vi "Example_LVQ.vi"() -> ()   [LabVIEW 2009]
uses:
  <vilib>/addons/Machine Learning/Utilities/Riffle (matrix with labels).vi
  <vilib>/addons/Machine Learning/NILabs_MLT.lvlib
panel:
  out "Data and learned centroids":cluster{"X":dbl[], "Y":dbl[]}[](graph)
  in  "# of samples":i32=1000
  in  "Parameters":cluster{"learning rate":dbl, "da":dbl}={"learning rate"=0.1, "da"=0.9}
  in  "stopping criteria":cluster{"tolarence":dbl, "max iterations":i32}={"tolarence"=1e-05, "max iterations"=50}
  in  "# of neurons":i32=16
  out "Time (ms)":u32
  # "Introduction:\nLearning Vector Quantization (LVQ) is used to learn the cluster structure of a data distrubution with four Gaussian centers."
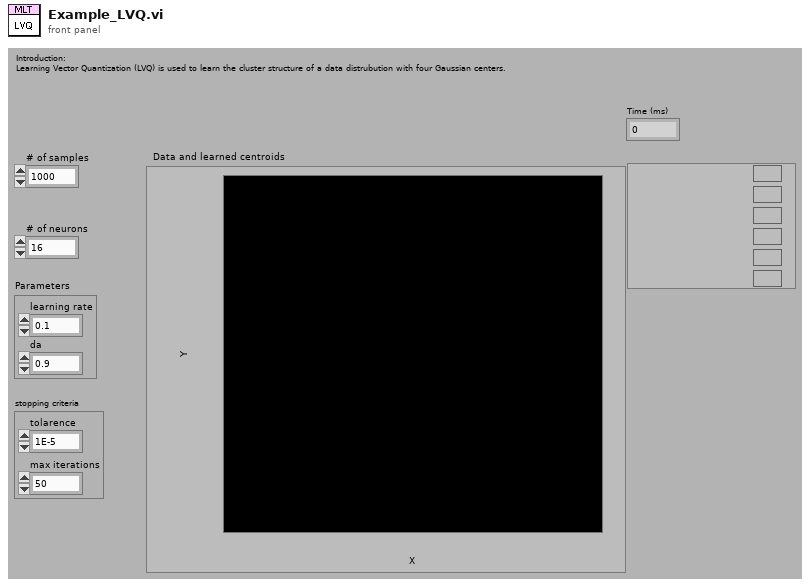
[diagram p1: front panel]
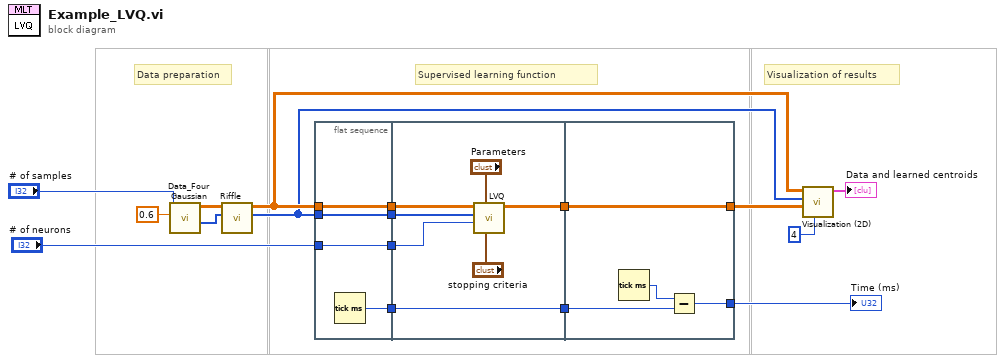
[diagram p0: block diagram]
diagram:
  # "Visualization of results"
  # "Supervised learning function"
  # "Data preparation"
  n1 = call "Data_Four Gaussian.vi"("noise amplitude"=0.6, "# of points"="# of samples") -> ("Classes"=w6:i32[], "Data"=w8:dbl[][])  [unwired: 8 in]
  n2 = call-poly <vilib>:"Riffle.vi"("Labels"=w6, "Data"=w8) -> ("Riffled{Labels}"=w5:i32[], "Riffled{Data}"=w7:dbl[][])  [unwired: 6 in, 2 out]
  n3 = flat-sequence {
    tunnel: [w21] -> w15
    tunnel: [w20] -> w13
    tunnel: w7 -> [w20]
    tunnel: w5 -> [w19]
    tunnel: [w19] -> w12
    tunnel: "# of neurons" -> [w18]
    tunnel: [w18] -> w2
    tunnel: [w28] -> w17
    tunnel: [w27] -> w16
    tunnel: w15 -> [w27]
    tunnel: w13 -> [w26]
    tunnel: w12 -> [w24]
    tunnel: w2 -> [w22]
    tunnel: [w32] -> w11
    tunnel: w17 -> [w32]
    tunnel: w16 -> [w31]
    tunnel: [w29] -> w14
    frame #0 {
      n4 = Tick Count (ms)() -> (millisecond timer value=w21:u32)
    }
    frame #1 {
      n5 = call <vilib>:"LVQ.vi"("Stopping criteria"="stopping criteria", "parameters"="Parameters", "# of neurons"=w22, "Class labels"=w24, "Data samples"=w26) -> ("Weights"=w28:dbl[][])  [unwired: 4 in, 2 out]
    }
    frame #2 {
      n6 = Tick Count (ms)() -> (millisecond timer value=w30:u32)
      n7 = Subtract(x=w30, y=w31) -> (x-y=w29:u32)
    }
  }
  n8 = call <vilib>:"Visualization (2D).vi"("# of classes"=4, "Centroids"=w11, "Class labels"=w5, "Data samples"=w7) -> ("XY Graph"=→"Data and learned centroids":cluster{"X":dbl[], "Y":dbl[]}[])  [unwired: 6 in, 1 out]
  "Time (ms)" <- w14
